vi "Extract Random variable-draw in chart - save file.vi"() -> ()   [LabVIEW 2018]
panel:
  out "웨이브폼 차트":dbl(graph)
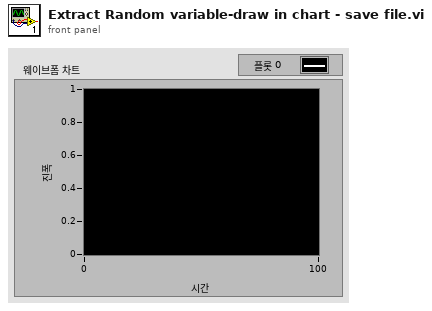
[diagram p1: front panel]
types:
  T1 = enum16{"open", "replace", "create", "open or create", "replace or create", "replace or create with confirmation"}
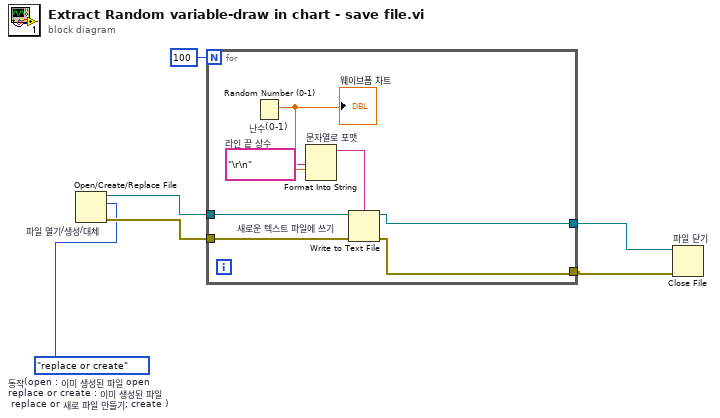
[diagram p0: block diagram]
diagram:
  w1 = T1."replace or create"  # 동작(open : 이미 생성된 파일 open replace or create : 이미 생성된 파일  replace or 새로 파일 만들기; create )
  n1 = Open/Create/Replace File "파일 열기/생성/대체"(operation (0:open)=w1) -> (refnum out=w5:refnum<file>, error out=w3:errorcluster)  [unwired: 5 in, 1 out]
  n2 = for {
    N: 100 -> [_]
    tunnel: w5 -> [w11]
    tunnel: [w10] -> w4
    tunnel: w3 -> [w9]
    tunnel: [w8] -> w2
    w12 = "\r\n"  # 라인 끝 상수
    n3 = Random Number (0-1) "난수(0-1)"() -> (number: 0 to 1=w13:dbl)
    "웨이브폼 차트" <- w13
    n4 = Format Into String "문자열로 포맷"(w13, w12) -> (resulting string=w7:string)  [unwired: 3 in, 1 out]
    n5 = Write to Text File "새로운 텍스트 파일에 쓰기"(file (use dialog)=w11, text=w7, error in=w9) -> (refnum out=w10:refnum<file>, error out=w8:errorcluster)  [unwired: 1 in, 1 out]
  }
  n6 = Close File "파일 닫기"(refnum=w4, error in=w2) -> ()  [unwired: 2 out]
